vi "DBGetData.vi"(8 "error in":errorcluster caption="错误输入", 10 "String":string, 11 "Procedure":string="prc_PackGetdata") -> (0 "error out":errorcluster, 1 "Data Out":string[][](array[string]))   [LabVIEW 2013]
uses:
  <vilib>/addons/database/Connection.llb/DB Tools Open Connec (String).vi
  <vilib>/addons/database/Connection.llb/Conn Execute.vi
  <vilib>/addons/database/Recordset.llb/Rec Fetch Recordset Data (R).vi
  <vilib>/addons/database/Recordset.llb/Rec Destroy - Connection.vi
  <vilib>/addons/database/NI_Database_API.lvlib
panel:
  out "子数组":string[](array[string])
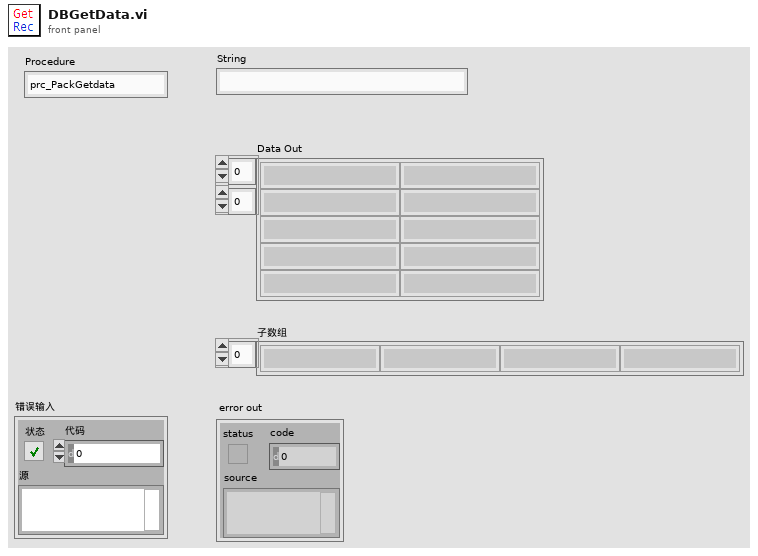
[diagram p1: front panel]
types:
  T1 = typedef "NI_Database_API.lvlib/Conn ObjectReference.ctl" = refnum<k1>
  T2 = typedef "NI_Database_API.lvlib/Rec ObjectReference.ctl" = refnum<k1>
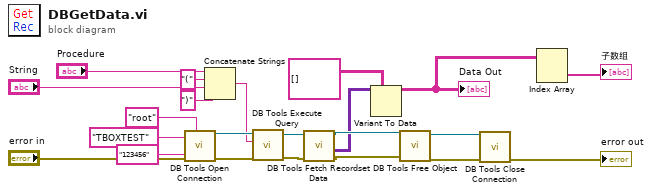
[diagram p0: block diagram]
diagram:
  n1 = call-poly <vilib>:"DB Tools Open Connection.vi"("password"="123456", "userID"="root", "error in (no error)"="error in", "connection information"="TBOXTEST" ("元素")) -> ("error out"=w19:errorcluster, "connection reference"=w20:T1)  [unwired: 4 in]
  n2 = Concatenate Strings("Procedure", "(" ("字符串"), "String", ")" ("字符串")) -> (w11:string)
  n3 = call-poly <vilib>:"DB Tools Execute Query.vi"("error in (no error)"=w19, "SQL query"=w11, "connection reference"=w20) -> ("error out"=w7:errorcluster, "recordset reference"=w8:T2)  [unwired: 5 in]
  n4 = call-poly <vilib>:"DB Tools Fetch Recordset Data.vi"("error in (no error)"=w7, "recordset reference"=w8) -> ("error out"=w6:errorcluster, "recordset data"=w4:variant[][], "recordset reference out"=w5:T2)  [unwired: 3 in]
  n5 = Variant To Data(type=string[][] [] ("数组"), Variant=w4) -> (data=w3:string[][])  [unwired: 1 in, 1 out]
  "Data Out" <- w3
  n6 = call-poly <vilib>:"DB Tools Free Object.vi"("error in (no error)"=w6, "recordset reference"=w5) -> ("error out"=w18:errorcluster, "connection reference"=w17:T1)  [unwired: 8 in]
  n7 = call <vilib>:"DB Tools Close Connection.vi"("error in (no error)"=w18, "connection reference"=w17) -> ("error out"=→"error out":errorcluster)  [unwired: 5 in]
  n8 = Index Array(array=w3) -> (element=→"子数组":string[])  [unwired: 2 in]
